vi "Protection.vi"(6 "OC protection":bool, 7 "OV protection":bool, 8 "error in (no error)":errorcluster, 10 "OV Value (10V)":dbl=10.0, 11 "VISA resource name":refnum<visa-resource-name>) -> (0 "error out":errorcluster, 3 "VISA resource name out":refnum<visa-resource-name>)   [LabVIEW 2017]
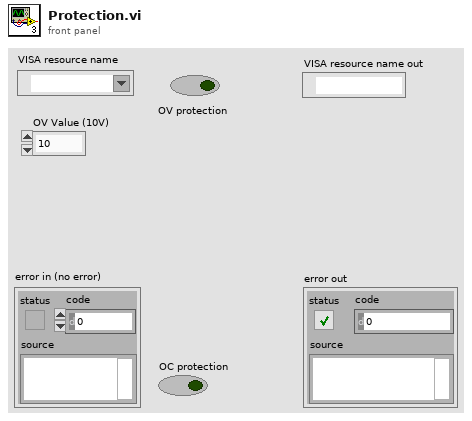
[diagram p1: front panel]
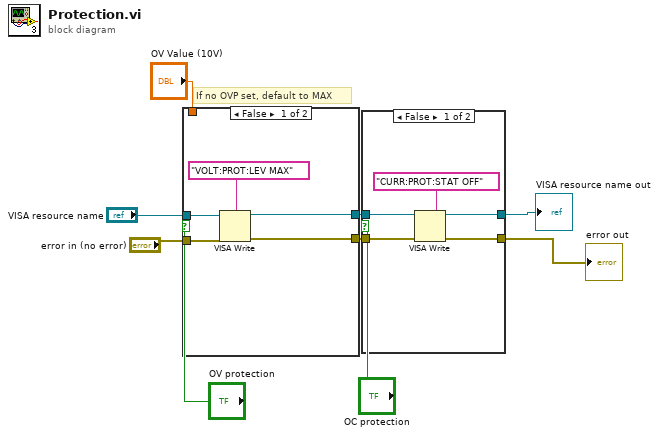
[diagram p0: block diagram]
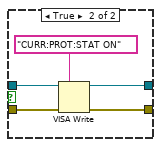
[diagram p2: hidden frame]
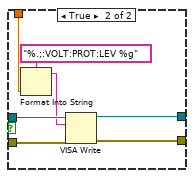
[diagram p3: hidden frame]
diagram:
  # "If no OVP set, default to MAX"
  n1 = case shown="False" "OV protection" {
    tunnel: "VISA resource name" -> [w14 w21]
    tunnel: "error in (no error)" -> [w13 w20]
    tunnel: [w11 w19] -> w7
    tunnel: [w12 w18] -> w6
    tunnel: "OV Value (10V)" -> [_ w15]
    frame False {
      n2 = VISA Write(VISA resource name=w14, write buffer="VOLT:PROT:LEV MAX", error in (no error)=w13) -> (VISA resource name out=w11:refnum<visa-resource-name>, error out=w12:errorcluster)  [unwired: 1 out]
    }
    frame True {
      n3 = Format Into String(format string="%.;:VOLT:PROT:LEV %g", w15) -> (resulting string=w16:string)  [unwired: 2 in, 1 out]
      n4 = VISA Write(VISA resource name=w21, write buffer=w16, error in (no error)=w20) -> (VISA resource name out=w19:refnum<visa-resource-name>, error out=w18:errorcluster)  [unwired: 1 out]
    }
  }
  n5 = case shown="False" "OC protection" {
    tunnel: w7 -> [w25 w31]
    tunnel: w6 -> [w24 w30]
    tunnel: [w23 w29] -> w1
    tunnel: [w22 w28] -> w2
    frame False {
      n6 = VISA Write(VISA resource name=w25, write buffer="CURR:PROT:STAT OFF", error in (no error)=w24) -> (VISA resource name out=w23:refnum<visa-resource-name>, error out=w22:errorcluster)  [unwired: 1 out]
    }
    frame True {
      n7 = VISA Write(VISA resource name=w31, write buffer="CURR:PROT:STAT ON", error in (no error)=w30) -> (VISA resource name out=w29:refnum<visa-resource-name>, error out=w28:errorcluster)  [unwired: 1 out]
    }
  }
  "error out" <- w2
  "VISA resource name out" <- w1
